vi "TemperatureRT.vi"(8 "error in (no error)":errorcluster) -> (0 "error out":errorcluster, 3 "TempArray":dbl[](array[numeric]))   [LabVIEW 2016]
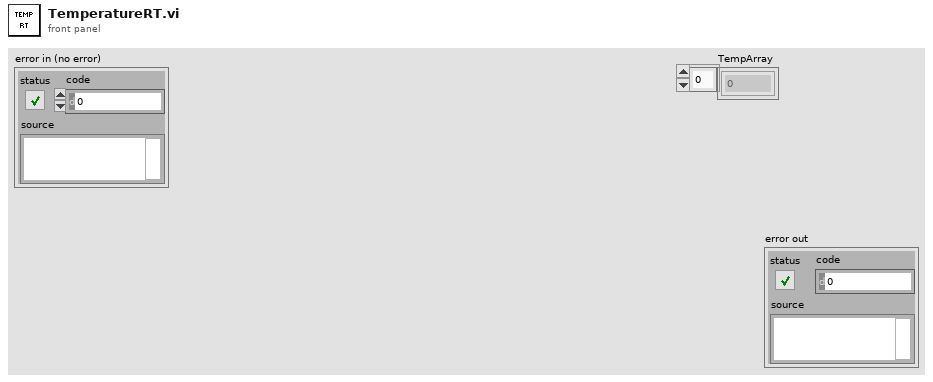
[diagram p1: front panel]
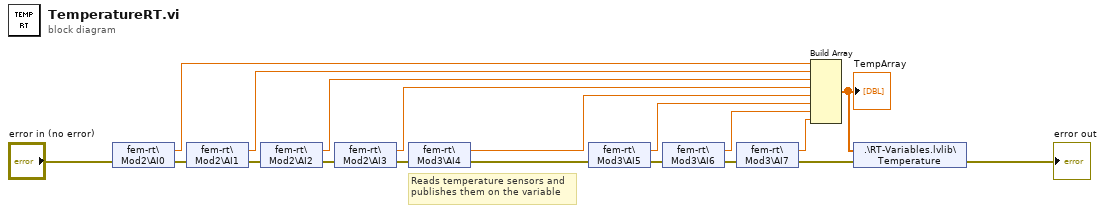
[diagram p0: block diagram]
diagram:
  # "Reads temperature sensors and\npublishes them on the variable"
  n1 = shared-variable "fem-rt\\Mod2\\AI0"(error in="error in (no error)") -> (w12:dbl, error out=w11:errorcluster)
  n2 = shared-variable "fem-rt\\Mod2\\AI1"(error in=w11) -> (w18:dbl, error out=w10:errorcluster)
  n3 = shared-variable "fem-rt\\Mod2\\AI2"(error in=w10) -> (w17:dbl, error out=w9:errorcluster)
  n4 = shared-variable "fem-rt\\Mod2\\AI3"(error in=w9) -> (w16:dbl, error out=w8:errorcluster)
  n5 = shared-variable "fem-rt\\Mod3\\AI4"(error in=w8) -> (w15:dbl, error out=w7:errorcluster)
  n6 = shared-variable "fem-rt\\Mod3\\AI5"(error in=w7) -> (w4:dbl, error out=w6:errorcluster)
  n7 = shared-variable "fem-rt\\Mod3\\AI6"(error in=w6) -> (w14:dbl, error out=w5:errorcluster)
  n8 = shared-variable "fem-rt\\Mod3\\AI7"(error in=w5) -> (w13:dbl, error out=w3:errorcluster)
  n9 = Build Array(w12, w18, w17, w16, w15, w4, w14, w13) -> (w1:dbl[])
  "TempArray" <- w1
  n10 = shared-variable ".\\RT-Variables.lvlib\\Temperature"(w1, error in=w3) -> (error out=→"error out":errorcluster)
